vi "BellMeasurement.vi"() -> ()   [LabVIEW 2018]
uses:
  <vilib>/Platform/TimedLoop/XDataNode/timing_clust.ctl
  <vilib>/Platform/TimedLoop/XDataNode/nitl_modes.ctl
  <vilib>/Platform/TimedLoop/XDataNode/wakeup.ctl
  <vilib>/rvi/Emulation/niFpgaSctlEmulationGetInTimedLoop.vi
  <vilib>/rvi/Emulation/niFpgaEmulationReportErrorSimple.vi
  <vilib>/rvi/Emulation/niFpgaGetClockAttributes.vi
  <vilib>/rvi/Emulation/niFpgaCriticalErrorInLSC.vi
  <vilib>/rvi/eio/common/nirviEmuTemplateMethod_errors.vi
  <vilib>/Platform/TimedLoop/XDataNode/XDataNode.xnode
  <vilib>/eio/EIONode/EIONode.xnode
  <vilib>/Platform/TimedLoop/XDataNode/XDNodeRunTimeDep.lvlib
panel:
  out "F-m":bool[](array[boolean])
  out "1H-m":bool[](array[boolean])
  out "1V-m":bool[](array[boolean])
  out "2H-m":bool[](array[boolean])
  out "Count":i16
  out "2V-m":bool[](array[boolean])
  out "04":i16
  out "03":i16
  out "02":i16
  out "01":i16
  out "clock2":i16
  out "14":i16
  out "13":i16
  out "12":i16
  out "1":i16
  out "Final":bool
  out "2V-ad":bool
  out "2H-ad":bool
  out "1V-ad":bool
  out "1H-ad":bool
  out "SE_Ch4_Rd":bool
  out "SE_Ch3_Rd":bool
  out "SE_Ch2_Rd":bool
  out "SE_Ch1_Rd":bool
  out "clock1":i16
  out "Test":bool
  in  "Probing-Depth":i16
  in  "Stop Button":bool
  in  "2V":i16
  in  "1V":i16
  in  "2H":i16
  in  "1H":i16
  out "Round":u32 format="%^.0e"
  # "OriginSignal"
  # "AfterDelay"
  # "Memory："
  # "DelaySetting："
  # "11"
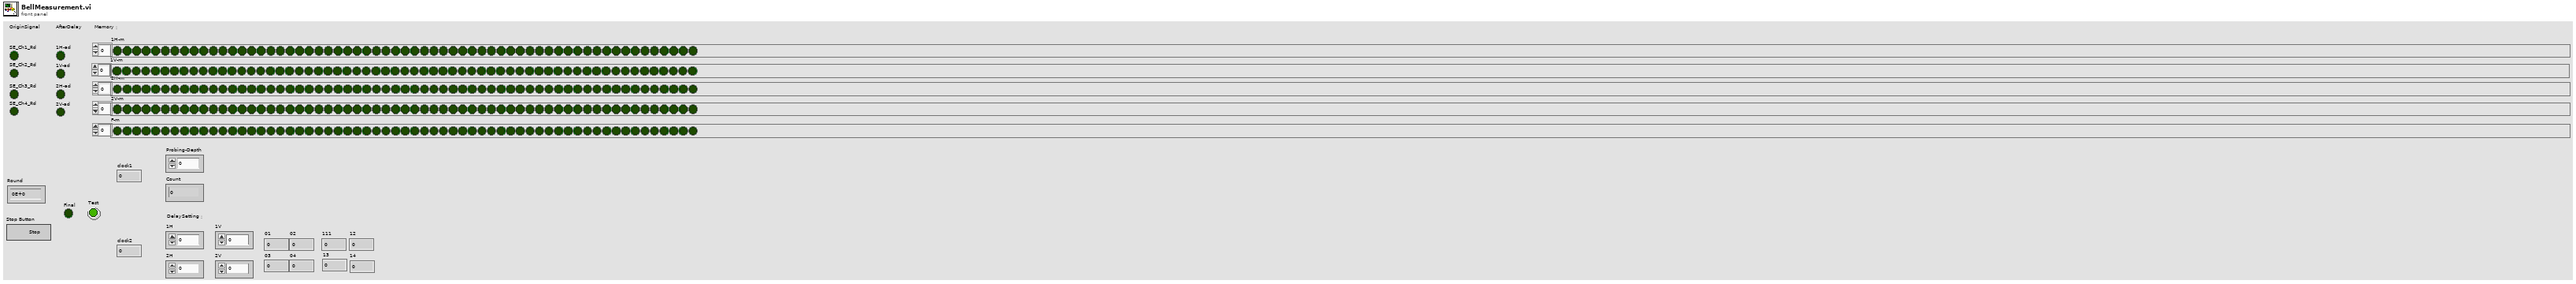
[diagram p1: front panel]
types:
  T1 = typedef "XDNodeRunTimeDep.lvlib/timing_clust.ctl" = cluster{"Expected End [f-1]":u64, "Actual End [f-1]":u64, "Finished Late? [f-1]":bool, "Expected End [i-1]":u64, "Actual End [i-1]":u64, "Finished Late? [i-1]":bool, "Expected Start [i]":u64, "Actual Start [i]":u64, "Expected Start [f]":u64, "Actual Start [f]":u64, "Source Name":string, "Structure Name":string, "Period":i64, "Deadline":i64, "Offset":i64, "Start":i64, "Priority":i32, "Timeout":i32, "Mode":T2, "Wakeup Reason":T3, "Error":errorcluster, "Source Type":string, "Secondary Source Type":string, "Global End Time":u64, "Global Start Time":u64, "Frame Duration":u64, "Iteration Duration":u64, "Assigned CPU":i32, "I/O Scan Engine Mode":u32}
  T2 = typedef "XDNodeRunTimeDep.lvlib/nitl_modes.ctl" = enum32{"No Change", "Process missed periods, maintain original phase", "Discard missed periods, maintain original phase", "Process missed periods, ignore original phase", "Discard missed periods, ignore original phase"}
  T3 = typedef "XDNodeRunTimeDep.lvlib/wakeup.ctl" = enum32{"Normal", "Aborted", "Asynchronous wakeup", "Timing source error", "Timed loop error", "Timeout"}
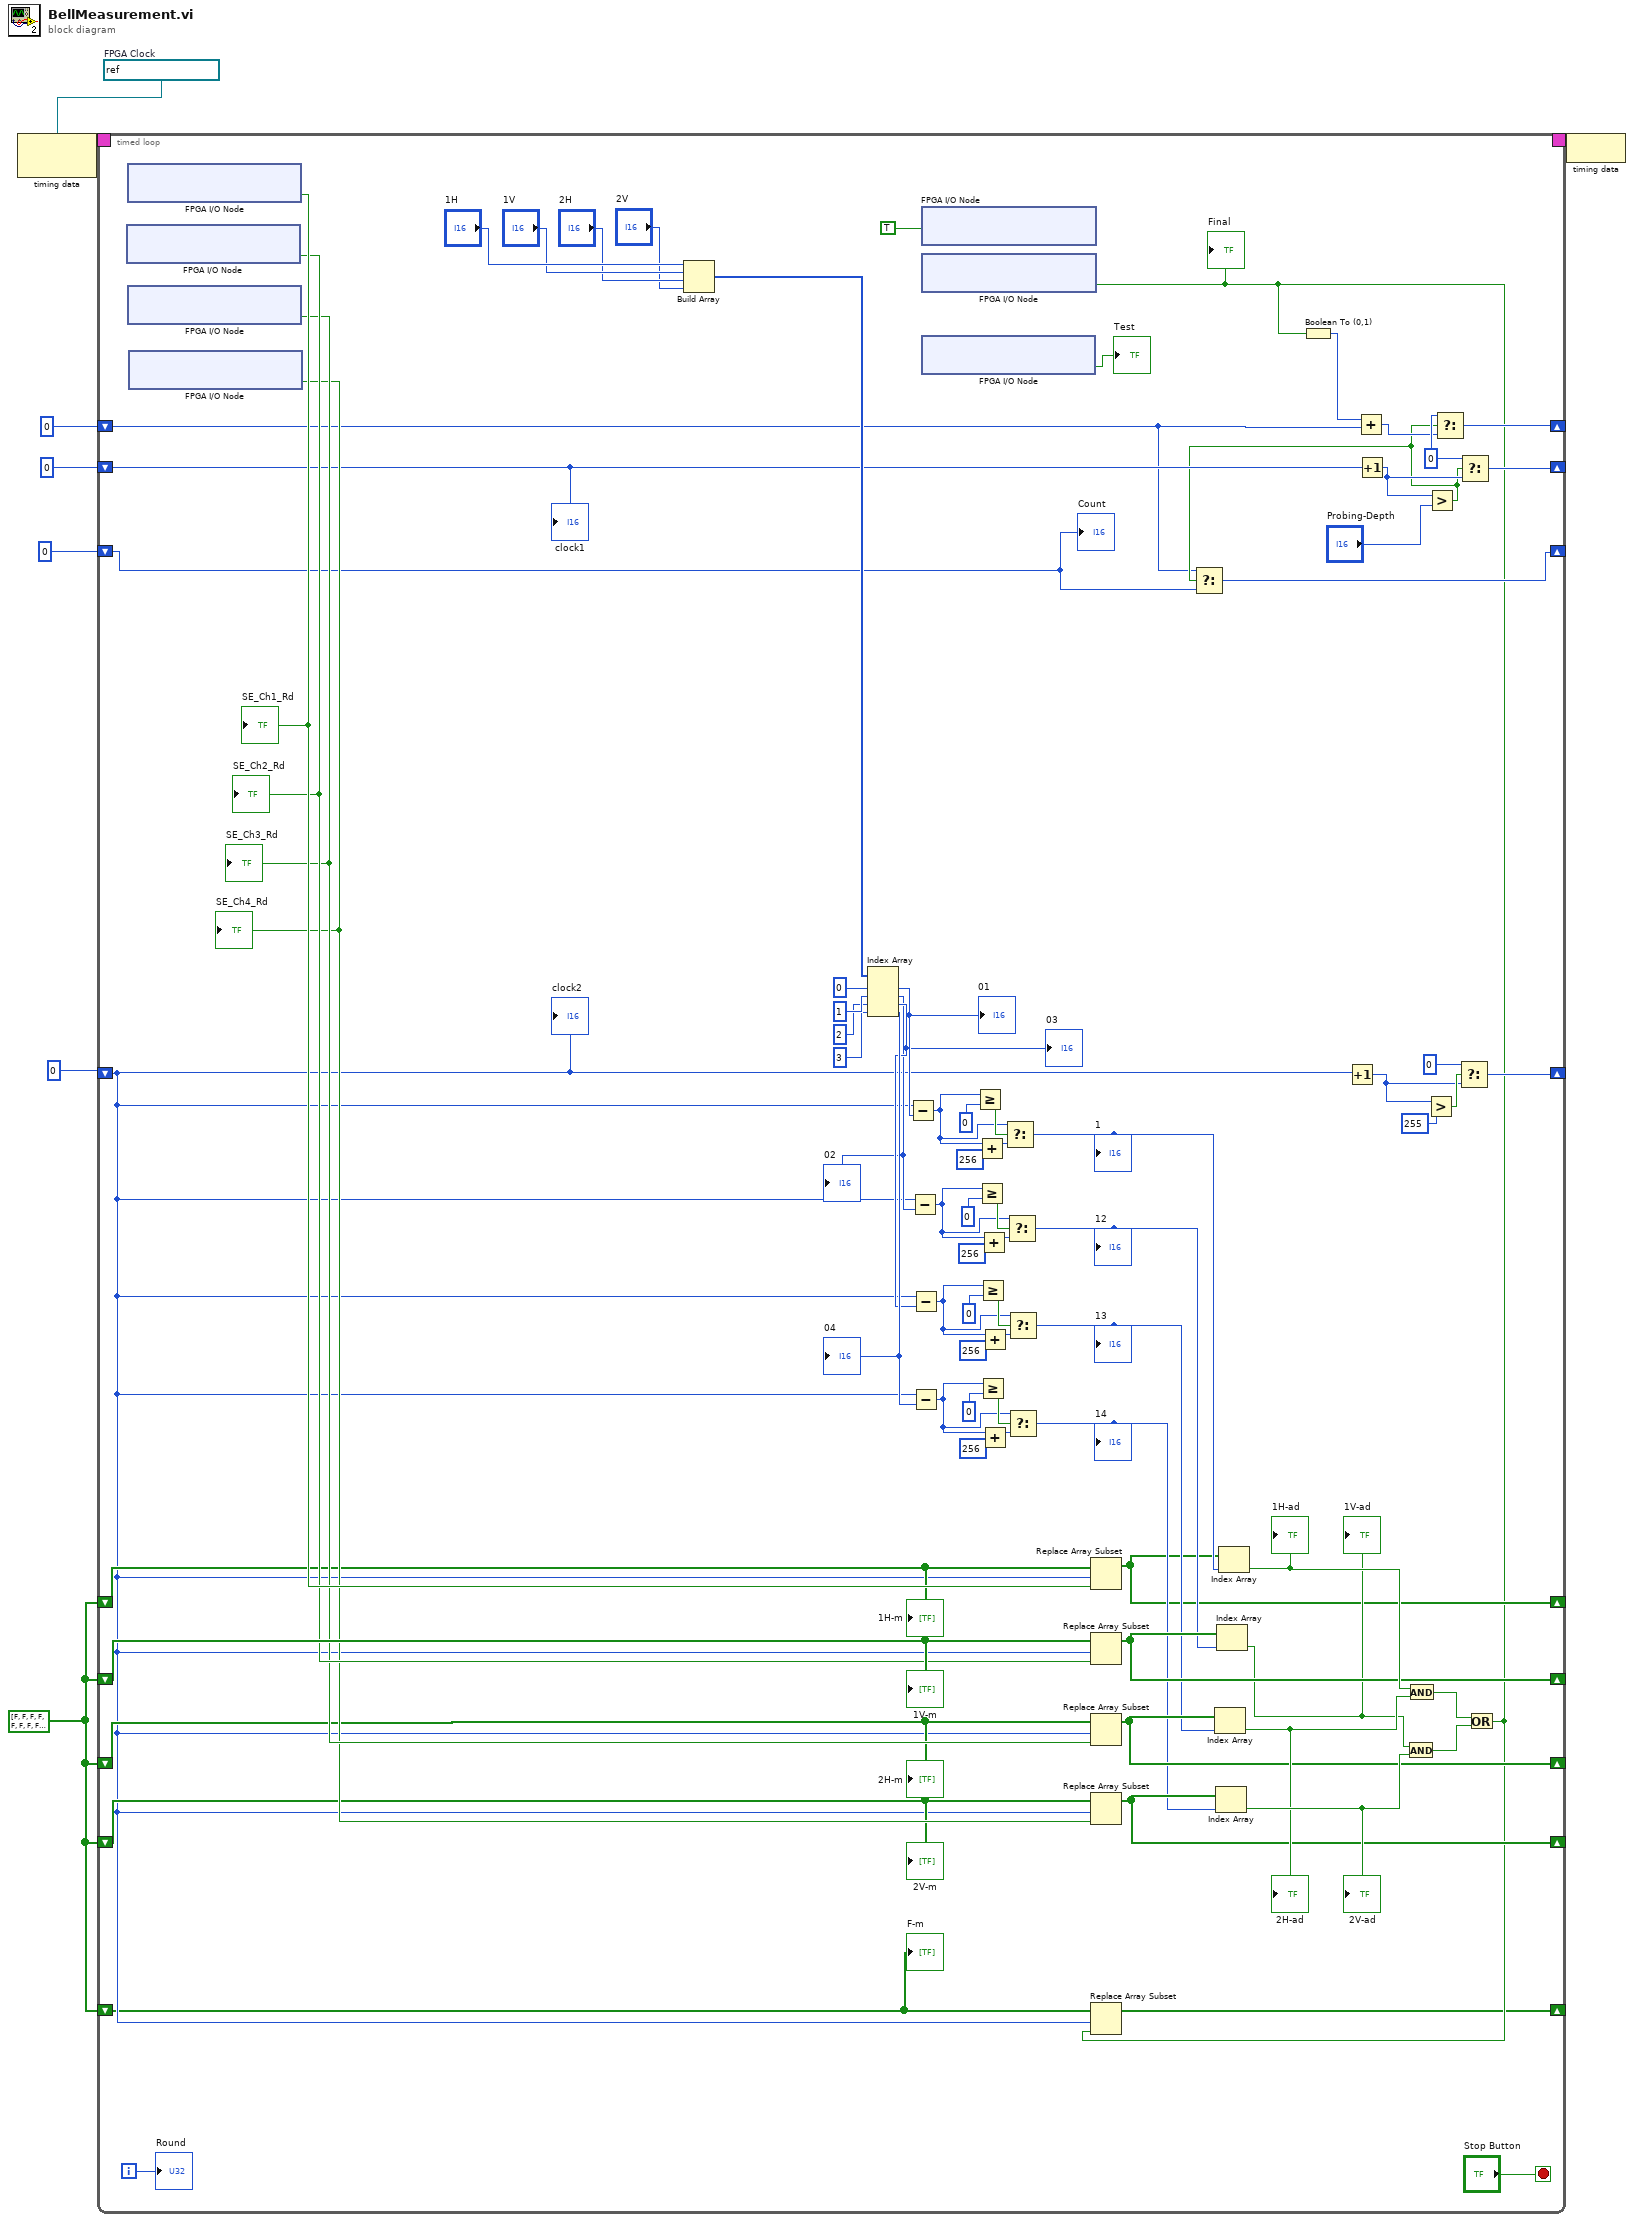
[diagram p0: block diagram]
diagram:
  w1 = bool[] [FALSE, FALSE, FALSE, FALSE, FALSE, FALSE, FALSE, FALSE, FALSE, FALSE, FALSE, FALSE, FALSE, FALSE, FALSE, FALSE, FALSE, FALSE, FALSE, FALSE, FALSE, FALSE, FALSE, FALSE, FALSE, FALSE, FALSE, FALSE, FALSE, FALSE, FALSE, FALSE, FALSE, FALSE, FALSE, FALSE, FALSE, FALSE, FALSE, FALSE, FALSE, FALSE, FALSE, FALSE, FALSE, FALSE, FALSE, FALSE, FALSE, FALSE, FALSE, FALSE, FALSE, FALSE, FALSE, FALSE, FALSE, FALSE, FALSE, FALSE, FALSE, FALSE, FALSE, FALSE, FALSE, FALSE, FALSE, FALSE, FALSE, FALSE, FALSE, FALSE, FALSE, FALSE, FALSE, FALSE, FALSE, FALSE, FALSE, FALSE, FALSE, FALSE, FALSE, FALSE, FALSE, FALSE, FALSE, FALSE, FALSE, FALSE, FALSE, FALSE, FALSE, FALSE, FALSE, FALSE, FALSE, FALSE, FALSE, FALSE, FALSE, FALSE, FALSE, FALSE, FALSE, FALSE, FALSE, FALSE, FALSE, FALSE, FALSE, FALSE, FALSE, FALSE, FALSE, FALSE, FALSE, FALSE, FALSE, FALSE, FALSE, FALSE, FALSE, FALSE, FALSE, FALSE, FALSE, FALSE, FALSE, FALSE, FALSE, FALSE, FALSE, FALSE, FALSE, FALSE, FALSE, FALSE, FALSE, FALSE, FALSE, FALSE, FALSE, FALSE, FALSE, FALSE, FALSE, FALSE, FALSE, FALSE, FALSE, FALSE, FALSE, FALSE, FALSE, FALSE, FALSE, FALSE, FALSE, FALSE, FALSE, FALSE, FALSE, FALSE, FALSE, FALSE, FALSE, FALSE, FALSE, FALSE, FALSE, FALSE, FALSE, FALSE, FALSE, FALSE, FALSE, FALSE, FALSE, FALSE, FALSE, FALSE, FALSE, FALSE, FALSE, FALSE, FALSE, FALSE, FALSE, FALSE, FALSE, FALSE, FALSE, FALSE, FALSE, FALSE, FALSE, FALSE, FALSE, FALSE, FALSE, FALSE, FALSE, FALSE, FALSE, FALSE, FALSE, FALSE, FALSE, FALSE, FALSE, FALSE, FALSE, FALSE, FALSE, FALSE, FALSE, FALSE, FALSE, FALSE, FALSE, FALSE, FALSE, FALSE, FALSE, FALSE, FALSE, FALSE, FALSE, FALSE, FALSE, FALSE, FALSE, FALSE, FALSE, FALSE, FALSE, FALSE, FALSE, FALSE, FALSE, FALSE, FALSE, FALSE, FALSE, FALSE, FALSE, FALSE, FALSE, FALSE, FALSE, FALSE, FALSE, FALSE, FALSE, FALSE]
  w6 = refnum<k21> "200 MHz Clock"  # FPGA Clock
  n1 = node-c288(w6) -> (w8:T1)
  n2 = timed-loop {
    timing: w8 -> [_]
    timing-out: [_] -> w7
    shift-right: [w22] -> _
    shift-left: w1 -> [w18]
    shift-right: [w75] -> _
    shift-left: w1 -> [w76]
    shift-right: [w73] -> _
    shift-left: w1 -> [w17]
    shift-right: [w71] -> _
    shift-left: w1 -> [w19]
    shift-right: [w77] -> _
    shift-left: i16 0 -> [w12]
    shift-right: [w35] -> _
    shift-left: i16 0 -> [w29]
    shift-right: [w30] -> _
    shift-left: i16 0 -> [w14]
    shift-right: [w15] -> _
    shift-left: i16 0 -> [w13]
    shift-right: [w10] -> _
    shift-left: w1 -> [w9]
    i -> [w85]
    stop <- "Stop Button" stop-if-true
    w32 = i16 0
    n3 = xnode "FPGA I/O Node"() -> ("IO Module\\SE_Ch2_Rd"=w74:bool)  [unwired: 1 in, 1 out]
    "SE_Ch2_Rd" <- w74
    n4 = xnode "FPGA I/O Node"() -> ("IO Module\\SE_Ch1_Rd"=w81:bool)  [unwired: 1 in, 1 out]
    "SE_Ch1_Rd" <- w81
    n5 = xnode "FPGA I/O Node"() -> ("IO Module\\SE_Ch3_Rd"=w72:bool)  [unwired: 1 in, 1 out]
    "SE_Ch3_Rd" <- w72
    n6 = xnode "FPGA I/O Node"() -> ("IO Module\\SE_Ch4_Rd"=w70:bool)  [unwired: 1 in, 1 out]
    "SE_Ch4_Rd" <- w70
    n7 = Build Array("1H", "1V", "2H", "2V") -> (w64:i16[])
    n8 = Index Array(array=w64, index #1=i16 0, index #2=i16 1, index #3=i16 2, index #4=i16 3) -> (element #1=w62:i16, element #2=w20:i16, element #3=w21:i16, element #4=w41:i16)
    "01" <- w62
    "02" <- w20
    "03" <- w21
    "04" <- w41
    n9 = Subtract(x=w12, y=w62) -> (x-y=w26:i16)
    n10 = Subtract(x=w12, y=w20) -> (x-y=w25:i16)
    n11 = Subtract(x=w12, y=w21) -> (x-y=w24:i16)
    n12 = Subtract(x=w12, y=w41) -> (x-y=w23:i16)
    n13 = xnode "FPGA I/O Node"("IO Module\\SE_Ch5_Dir"=TRUE) -> ()  [unwired: 1 in, 1 out]
    n14 = xnode "FPGA I/O Node"() -> ("IO Module\\SE_Ch6_Rd"=→"Test":bool)  [unwired: 1 in, 1 out]
    n15 = Greater Or Equal?(x=w26, y=i16 0) -> (x >= y?=w58:bool)
    n16 = Add(x=w26, y=i16 256) -> (x+y=w60:i16)
    n17 = Greater Or Equal?(x=w25, y=i16 0) -> (x >= y?=w51:bool)
    n18 = Greater Or Equal?(x=w24, y=i16 0) -> (x >= y?=w47:bool)
    n19 = Greater Or Equal?(x=w23, y=i16 0) -> (x >= y?=w43:bool)
    n20 = Add(x=w25, y=i16 256) -> (x+y=w53:i16)
    n21 = Add(x=w24, y=i16 256) -> (x+y=w49:i16)
    n22 = Add(x=w23, y=i16 256) -> (x+y=w45:i16)
    n23 = Select(t=w26, s=w58, f=w60) -> (s? t:f=w61:i16)
    "1" <- w61
    n24 = Select(t=w25, s=w51, f=w53) -> (s? t:f=w39:i16)
    "12" <- w39
    n25 = Select(t=w24, s=w47, f=w49) -> (s? t:f=w40:i16)
    "13" <- w40
    n26 = Select(t=w23, s=w43, f=w45) -> (s? t:f=w38:i16)
    "14" <- w38
    n27 = Replace Array Subset(array=w18, new element=w81, index=w12) -> (w22:bool[])
    n28 = Replace Array Subset(array=w76, new element=w74, index=w12) -> (w75:bool[])
    n29 = Replace Array Subset(array=w17, new element=w72, index=w12) -> (w73:bool[])
    n30 = Replace Array Subset(array=w19, new element=w70, index=w12) -> (w71:bool[])
    n31 = Index Array(array=w73, index=w40) -> (element=w82:bool)
    "2H-ad" <- w82
    n32 = Index Array(array=w71, index=w38) -> (element=w83:bool)
    "2V-ad" <- w83
    n33 = Index Array(array=w75, index=w39) -> (element=w27:bool)
    "1V-ad" <- w27
    n34 = Index Array(array=w22, index=w61) -> (element=w84:bool)
    "1H-ad" <- w84
    n35 = Increment(x=w12) -> (x+1=w69:i16)
    n36 = Increment(x=w29) -> (x+1=w36:i16)
    n37 = And(x=w27, y=w83) -> (x .and. y?=w87:bool)
    n38 = And(x=w84, y=w82) -> (x .and. y?=w88:bool)
    n39 = Greater?(x=w69, y=i16 255) -> (0:w79:bool)
    n40 = Greater?(x=w36, y="Probing-Depth") -> (0:w16:bool)
    n41 = Select(t=w14, s=w16, f=w13) -> (s? t:f=w15:i16)
    n42 = Select(t=i16 0, s=w79, f=w69) -> (s? t:f=w77:i16)
    n43 = Select(t=w32, s=w16, f=w36) -> (s? t:f=w35:i16)
    n44 = Or(x=w88, y=w87) -> (x .or. y?=w11:bool)
    "Final" <- w11
    n45 = xnode "FPGA I/O Node"("IO Module\\SE_Ch5_Wr"=w11) -> ()  [unwired: 1 in, 1 out]
    n46 = Replace Array Subset(array=w9, new element=w11, index=w12) -> (w10:bool[])
    n47 = Boolean To (0,1)(Boolean=w11) -> (0, 1=w33:i16)
    n48 = Add(x=w33, y=w14) -> (x+y=w31:i16)
    n49 = Select(t=w32, s=w16, f=w31) -> (s? t:f=w30:i16)
    "Round" <- w85
    "clock1" <- w29
    "clock2" <- w12
    "2V-m" <- w19
    "Count" <- w13
    "2H-m" <- w17
    "1V-m" <- w76
    "1H-m" <- w18
    "F-m" <- w9
  }
  n50 = node-c288(w7) -> ()
